vi "初始化程序.vi"(11 "棋盘大小":i32=15) -> (2 "当前棋盘状态":i32[][](array[numeric]), 3 "控制数组":bool[][](array[boolean]))   [LabVIEW 2018]
doc: "将棋盘恢复为空白的棋盘，同时将控制按钮的数组恢复为初始状态"
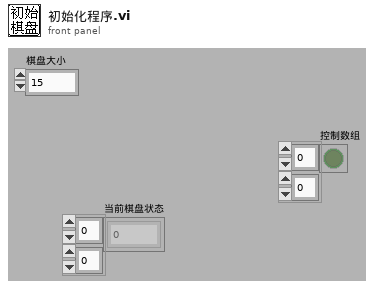
[diagram p1: front panel]
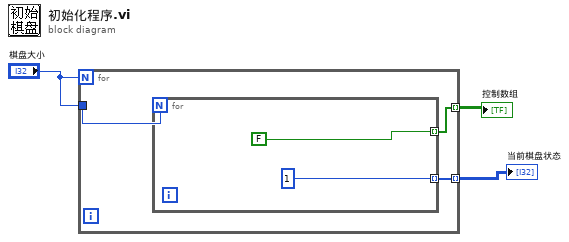
[diagram p0: block diagram]
diagram:
  n1 = for {
    N: "棋盘大小" -> [_]
    tunnel: [w6] -> w3 mode=indexing
    tunnel: "棋盘大小" -> [w5]
    tunnel: [w4] -> w1 mode=indexing
    n2 = for {
      N: w5 -> [_]
      tunnel: [FALSE] -> w6 mode=indexing
      tunnel: [1] -> w4 mode=indexing
    }
  }
  "当前棋盘状态" <- w1
  "控制数组" <- w3
